vi "AlliGator Get ICCD Information.vi"(5 "Y Resolution":i32, 7 "X Resolution":i32, 8 "Error In":errorcluster, 9 "Y Software Binning":i32, 10 "X Software Binning":i32, 11 "File Info":variant) -> (0 "Error Out":errorcluster, 3 "ICCD-specific Information":T1)   [LabVIEW 2021, in "AlliGator Files.lvlib"]
uses:
  AlliGator Files.lvlib
  AlliGator ICCD-specific Information.ctl
  AlliGator Image Folder Loading Information.ctl
  AlliGator RecSettings Metadata.ctl
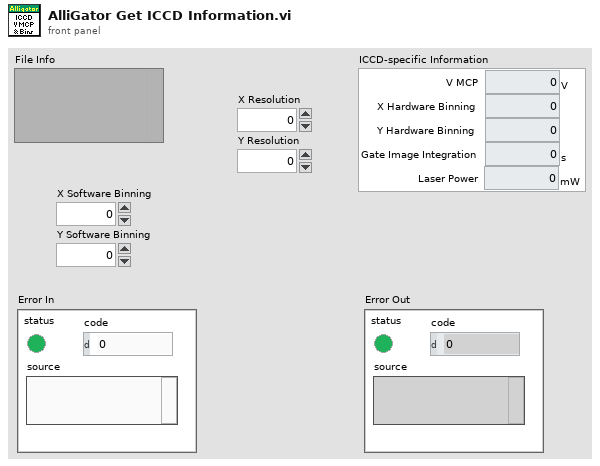
[diagram p1: front panel]
types:
  T1 = typedef "AlliGator Files.lvlib/AlliGator ICCD-specific Information.ctl" = cluster{"V MCP":dbl[unit], "X Hardware Binning":dbl, "Y Hardware Binning":dbl, "Gate Image Integration":dbl[unit], "Laser Power":dbl[unit]}
  T2 = typedef "AlliGator Files.lvlib/AlliGator Image Folder Loading Information.ctl" = cluster{"Image Folder":path, "Metadata":T3}
  T3 = typedef "AlliGator Files.lvlib/AlliGator RecSettings Metadata.ctl" = cluster{"Time Stamp (s)":dbl, "First Gate":dbl[unit], "Gate Step":dbl[unit], "# Gates":i32, "Gate Duration":dbl[unit], "Laser Period":dbl[unit], "Gate Image Integration":dbl[unit], "Date":timestamp, "V MCP":dbl[unit], "Binning":dbl}
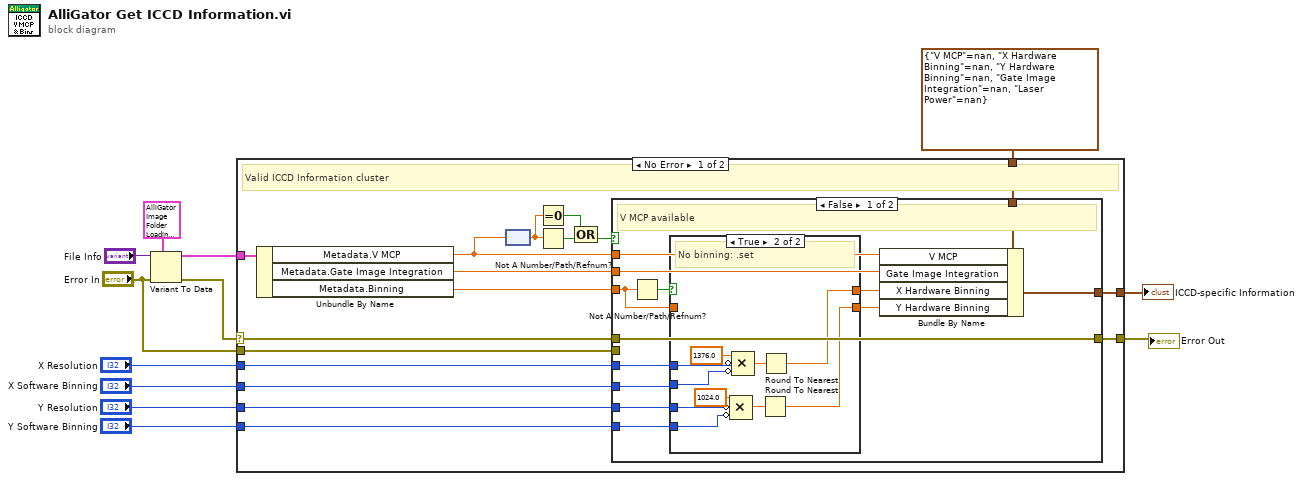
[diagram p0: block diagram]
diagram:
  n1 = Variant To Data(error in="Error In", type=T2 {"Image Folder"=path "", "Metadata"={"Time Stamp (s)"=0.0, "First Gate"=0.0, "Gate Step"=0.0, "# Gates"=0, "Gate Duration"=0.0, "Laser Period"=0.0, "Gate Image Integration"=0.0, "Date"=timestamp(0 s since 1904-01-01), "V MCP"=0.0, "Binning"=0.0}} ("Image Folder Loading Information"), Variant="File Info") -> (data=w11:T2, error out=w7:errorcluster)
  n2 = case shown="No Error" w7 {
    selector: w7 -> [w23 _]
    tunnel: w11 -> [w29 _]
    tunnel: T1 {"V MCP"=nan, "X Hardware Binning"=nan, "Y Hardware Binning"=nan, "Gate Image Integration"=nan, "Laser Power"=nan} ("ICCD-specific Information") -> [w28 w57]
    tunnel: [w27 w57] -> w8
    tunnel: [w19 w56] -> w6
    tunnel: "Error In" -> [w17 w56]
    tunnel: "X Resolution" -> [w16 _]
    tunnel: "X Software Binning" -> [w15 _]
    tunnel: "Y Resolution" -> [w14 _]
    tunnel: "Y Software Binning" -> [w13 _]
    frame No Error {
      # "Valid ICCD Information cluster"
      n3 = Unbundle By Name(w29) -> ("Metadata.V MCP"=w25:dbl[unit], "Metadata.Gate Image Integration"=w26:dbl[unit], "Metadata.Binning"=w18:dbl)
      n4 = node(w25) -> (w21:dbl)
      n5 = Equal To 0?(x=w21) -> (x = 0?=w20:bool)
      n6 = Not A Number/Path/Refnum?(number/path/refnum=w21) -> (NaN/Path/Refnum?=w24:bool)
      n7 = Compound Arithmetic op=OR(w20, w24) -> (w22:bool)
      n8 = case shown="False" w22 {
        tunnel: w28 -> [w42 w55]
        tunnel: [w41 w55] -> w27
        tunnel: w26 -> [w40 _]
        tunnel: w25 -> [w39 _]
        tunnel: w23 -> [w38 _]
        tunnel: [w38 w54] -> w19
        tunnel: w18 -> [w36 _]
        tunnel: w17 -> [_ w54]
        tunnel: w16 -> [w33 _]
        tunnel: w15 -> [w32 _]
        tunnel: w14 -> [w31 _]
        tunnel: w13 -> [w30 _]
        frame False {
          # "V MCP available"
          n9 = Not A Number/Path/Refnum?(number/path/refnum=w36) -> (NaN/Path/Refnum?=w37:bool)
          n10 = case shown="True" w37 {
            tunnel: w36 -> [w43 _]
            tunnel: [w43 w45] -> w35
            tunnel: [w43 w47] -> w34
            tunnel: w33 -> [_ w53]
            tunnel: w32 -> [_ w52]
            tunnel: w31 -> [_ w51]
            tunnel: w30 -> [_ w50]
            frame False {
              # "1040"
              # "1392"
              # "Binning: .txt"
            }
            frame True {
              # "No binning: .set"
              n11 = Compound Arithmetic op=MULTIPLY(1024.0 ("value"), invert w51, invert w50) -> (w46:dbl)
              n12 = Compound Arithmetic op=MULTIPLY(1376.0 ("value"), invert w53, invert w52) -> (w48:dbl)
              n13 = Round To Nearest(number=w46) -> (nearest integer value=w45:dbl)
              n14 = Round To Nearest(number=w48) -> (nearest integer value=w47:dbl)
            }
          }
          n15 = Bundle By Name(cluster=w42, "V MCP"=w39, "Gate Image Integration"=w40, "X Hardware Binning"=w34, "Y Hardware Binning"=w35) -> (w41:T1)
        }
        frame True {
          # "No V MCP: not a valid ICCD info"
        }
      }
    }
    frame Error {
    }
  }
  "ICCD-specific Information" <- w8
  "Error Out" <- w6
